vi "Z_3D_to_mouse_scroll.vi"(10 "Z":dbl) -> (2 "Scrolling":i32)   [LabVIEW 2011]
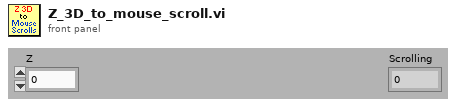
[diagram p1: front panel]
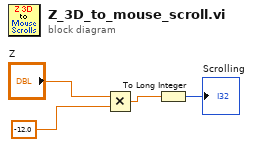
[diagram p0: block diagram]
diagram:
  n1 = Multiply(x="Z", y=-12.0) -> (x*y=w2:dbl)
  n2 = To Long Integer(number=w2) -> (32bit integer=→"Scrolling":i32)
